vi "Keithley 24XX Test and Memory Sweep.vi"() -> ()   [LabVIEW 2022 SP3]
doc: "This example creates two instrument setups in memory and sweeps through them depending on the results of a compliance test."
uses:
  Keithley 24XX.lvlib
  Initialize Folder/D/Download/Keithley 24XX/Public/Data/Low Level/Fetch (Measurements).vi
panel:
  out "Resistance":sgl[](array[numeric])
  out "Current":sgl[](array[numeric])
  out "Voltage":sgl[](array[numeric])
  in  "VISA resource name":refnum<visa-resource-name>
  in  "Serial Configuration":T1={"Baud Rate"=9600, "Parity"=0, "Data Bits"=8, "Stop Bits"=10, "Flow Control"=0} {"Flow Control" items=["None", "XON/XOFF", "RTS/CTS", "XON/XOFF & RTS/CTS", "DTR/DSR", "XON/XOFF & DTR/DSR"]; "Stop Bits" items=["1.0"=10, "1.5"=15, "2.0"=20]; "Data Bits" items=["7"=7, "8"=8]; "Parity" items=["None", "Odd", "Even", "Mark", "Space"]; "Baud Rate" items=["300"=300, "600"=600, "1200"=1200, "2400"=2400, "4800"=4800, "9600"=9600, "19200"=19200]}
  # "(c) 2006 - 2015 National Instruments.  ALL RIGHTS RESERVED."
  # "Note: The test values on the block diagram may need to be changed based on your DUT.  Please see the block diagram to check this as well as see how testing and memory sweeping are accomplished."
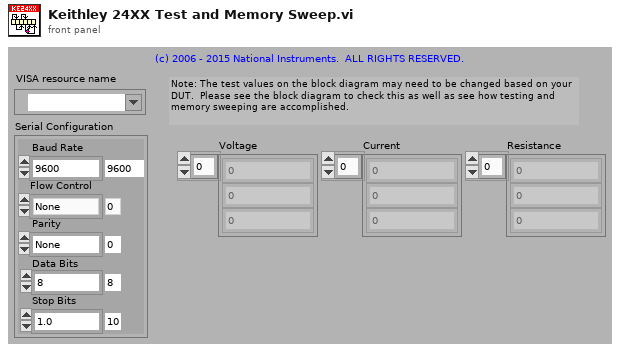
[diagram p1: front panel]
types:
  T1 = cluster{"Baud Rate":u32, "Parity":u16, "Data Bits":u16, "Stop Bits":u16, "Flow Control":u16}
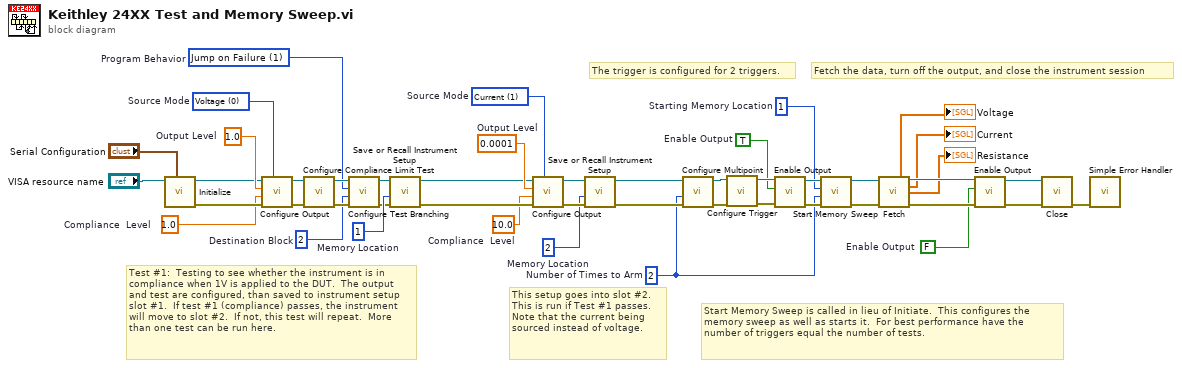
[diagram p0: block diagram]
diagram:
  w1 = u16 1 items=["Voltage", "Current"]  # Source Mode
  w2 = u16 0 items=["Voltage", "Current"]  # Source Mode
  w3 = 1.0  # Compliance  Level
  w4 = TRUE  # Enable Output
  w5 = FALSE  # Enable Output
  w6 = 10.0  # Compliance  Level
  w7 = u32 1  # Starting Memory Location
  w9 = u16 1 items=["Jump on Pass", "Jump on Failure", "Don't Jump"]  # Program Behavior
  w10 = u32 2  # Destination Block
  w8 = 2  # Number of Times to Arm
  w36 = u32 2  # Memory Location
  w37 = u32 1  # Memory Location
  w42 = 0.0001  # Output Level
  w43 = 1.0  # Output Level
  # "Fetch the data, turn off the output, and close the instrument session"
  # "Start Memory Sweep is called in lieu of Initiate.  This configures the memory sweep as well as starts it.  For best performance have the number of triggers equal the number of tests."
  # "The trigger is configured for 2 triggers."
  # "This setup goes into slot #2.  This is run if Test #1 passes.  Note that the current being sourced instead of voltage."
  # "Test #1:  Testing to see whether the instrument is in compliance when 1V is applied to the DUT.  The output and test are configured, than saved to instrument setup slot #1.  If test #1 (compliance) passes, the instrument will move to slot #2.  If not, this test will repeat.  More than one test can be run here."
  n1 = call "Initialize.vi"("Serial Configuration"="Serial Configuration", "VISA resource name"="VISA resource name") -> ("error out"=w32:errorcluster, "VISA resource name out"=w33:refnum<visa-resource-name>)  [unwired: 8 in]
  n2 = call "Configure Output.vi"("Source Mode  (0: Voltage)"=w2, "error in (no error)"=w32, "Compliance  Level (0.1)"=w3, "Output Level (0)"=w43, "VISA resource name"=w33) -> ("error out"=w15:errorcluster, "VISA resource name out"=w16:refnum<visa-resource-name>)  [unwired: 5 in]
  n3 = call "Configure Compliance Limit Test.vi"("error in (no error)"=w15, "VISA resource name"=w16) -> ("error out"=w13:errorcluster, "VISA resource name out"=w14:refnum<visa-resource-name>)  [unwired: 8 in]
  n4 = call "Configure Test Branching.vi"("error in (no error)"=w13, "Destination Block (1)"=w10, "Program Behavior (0: Jump on Pass)"=w9, "VISA resource name"=w14) -> ("error out"=w11:errorcluster, "VISA resource name out"=w12:refnum<visa-resource-name>)  [unwired: 6 in]
  n5 = call "Save or Recall Instrument Setup.vi"("error in (no error)"=w11, "Memory Location (1)"=w37, "VISA resource name"=w12) -> ("error out"=w34:errorcluster, "VISA resource name out"=w35:refnum<visa-resource-name>)  [unwired: 7 in]
  n6 = call "Configure Output.vi"("Source Mode  (0: Voltage)"=w1, "error in (no error)"=w34, "Compliance  Level (0.1)"=w6, "Output Level (0)"=w42, "VISA resource name"=w35) -> ("error out"=w40:errorcluster, "VISA resource name out"=w41:refnum<visa-resource-name>)  [unwired: 5 in]
  n7 = call "Save or Recall Instrument Setup.vi"("error in (no error)"=w40, "Memory Location (1)"=w36, "VISA resource name"=w41) -> ("error out"=w21:errorcluster, "VISA resource name out"=w22:refnum<visa-resource-name>)  [unwired: 7 in]
  n8 = call "Configure Multipoint.vi"("error in (no error)"=w21, "Trigger Count (1)"=w8, "VISA resource name"=w22) -> ("error out"=w19:errorcluster, "VISA resource name out"=w20:refnum<visa-resource-name>)  [unwired: 7 in]
  n9 = call "Configure Trigger.vi"("error in (no error)"=w19, "VISA resource name"=w20) -> ("error out"=w18:errorcluster, "VISA resource name out"=w17:refnum<visa-resource-name>)  [unwired: 8 in]
  n10 = call "Enable Output.vi"("error in (no error)"=w18, "Enable Output (T: Enable)"=w4, "VISA resource name"=w17) -> ("error out"=w39:errorcluster, "VISA resource name out"=w38:refnum<visa-resource-name>)  [unwired: 7 in]
  n11 = call "Start Memory Sweep.vi"("error in (no error)"=w39, "Number of Points (5)"=w8, "Starting Memory Location (1)"=w7, "VISA resource name"=w38) -> ("error out"=w28:errorcluster, "VISA resource name out"=w29:refnum<visa-resource-name>)  [unwired: 6 in]
  n12 = call-poly "Fetch.vi"("VISA resource name"=w29, "error in (no error)"=w28) -> ("Voltage"=→"Voltage":sgl[], "VISA resource name out"=w26:refnum<visa-resource-name>, "Current"=→"Current":sgl[], "Resistance"=→"Resistance":sgl[], "error out"=w27:errorcluster)  [unwired: 7 in, 2 out]
  n13 = call "Enable Output.vi"("error in (no error)"=w27, "Enable Output (T: Enable)"=w5, "VISA resource name"=w26) -> ("error out"=w30:errorcluster, "VISA resource name out"=w31:refnum<visa-resource-name>)  [unwired: 7 in]
  n14 = call "Close.vi"("error in (no error)"=w30, "VISA resource name"=w31) -> ("error out"=w44:errorcluster)  [unwired: 9 in]
  n15 = call <vilib>:"Simple Error Handler.vi"("error in (no error)"=w44) -> ()  [unwired: 4 in, 5 out]
